vi "GT Set Memory.vi"(7 "pData":i16, 8 "error in (no error)":errorcluster caption="错误输入（无错误）", 9 "count":i16, 10 "address":u32, 11 "cardNum":i16) -> (0 "error out":errorcluster caption="错误输出", 3 "function return":i16, 5 "pData out":i16)   [LabVIEW 2020, in "gts1.lvlib"]
doc: "GT_API GT_SetMemory(short cardNum,unsigned long address,short count,short *pData);"
uses:
  gts1.lvlib
  dll/32bit/multi_card/gts.dll
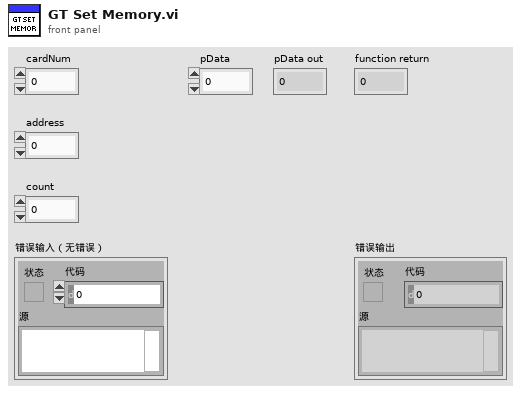
[diagram p1: front panel]
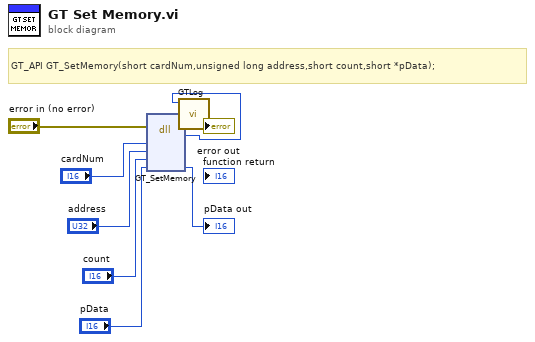
[diagram p0: block diagram]
diagram:
  # "GT_API GT_SetMemory(short cardNum,unsigned long address,short count,short *pData);"
  n1 = dll-call lib="C:/1228/dll/32bit/multi_card/gts.dll" fn="GT_SetMemory"(error in="error in (no error)", "cardNum"="cardNum", "address"="address", "count"="count", "pData"="pData") -> (error out=w3:errorcluster, w1:i16, "pData"=→"pData out":i16)  [unwired: 5 in, 1 out]
  n2 = call "GTLog.vi"("error in (no error)"=w3, "Numeric"=w1) -> ("error out"=→"error out":errorcluster)  [unwired: 9 in]
